vi "Test.vi"() -> ()   [LabVIEW 2018]
uses:
  Timer.lvclass
  Timer.lvclass/Timer.ctl
panel:
  out "Start Time":dbl
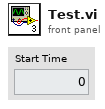
[diagram p1: front panel]
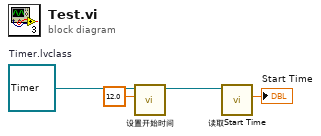
[diagram p0: block diagram]
diagram:
  w4 = refnum<class "Timer.lvclass"> refnum  # Timer.lvclass
  n1 = call-dynamic "设置开始时间.vi"("Start Time"=12.0, "Timer 输入"=w4) -> ("Timer 输出"=w2:refnum<class "Timer.lvclass">)  [unwired: 8 in, 1 out]
  n2 = call "读取Start Time.vi"("Timer输入"=w2) -> ("Start Time"=→"Start Time":dbl)  [unwired: 8 in, 2 out]
